vi "Add Pattern Script Header.vi"(8 "error in (no error)":errorcluster, 9 "Pattern Script Frame in":string, 10 "Pattern Name":string, 11 "SPI 4W Pattern Creator in":refnum<class "SPI 4W Pattern Creator.lvclass">) -> (0 "error out":errorcluster, 2 "Pattern Script All out":string, 3 "SPI 4W Pattern Creator out":refnum<class "SPI 4W Pattern Creator.lvclass">)   [LabVIEW 2018, in "SPI 4W Pattern Creator.lvlib" / "SPI 4W Pattern Creator.lvclass"]
uses:
  SPI 4W Pattern Creator.lvclass
  Interfaces/Protocol Interface.lvlibp/Interfaces/Protocol Interface/Pin State.ctl
  Interfaces/Protocol Interface.lvlibp/Interfaces/Protocol Interface/Protocol Interface.lvclass
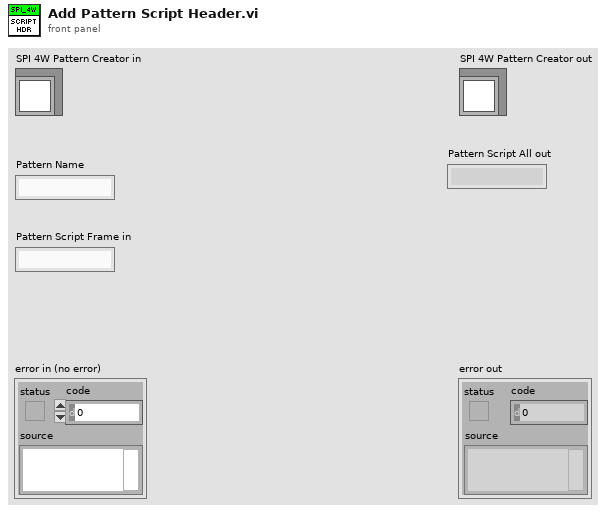
[diagram p1: front panel]
types:
  T1 = typedef "Protocol Interface.lvlibp/Protocol Interface.lvclass/Pin State.ctl" = enum16{"0", "1", "L", "H", "X", "V", "D", "M"}
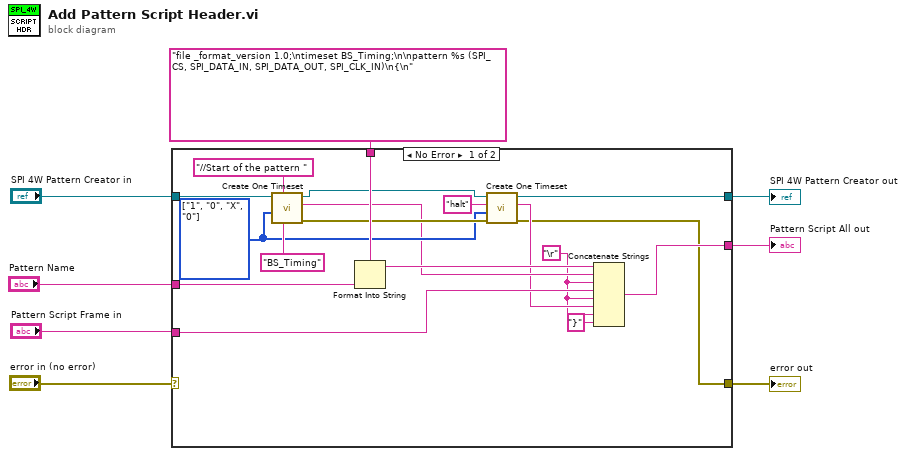
[diagram p0: block diagram]
diagram:
  n1 = case shown="No Error" "error in (no error)" {
    selector: "error in (no error)" -> [_ w28]
    tunnel: "Pattern Name" -> [w26 _]
    tunnel: "file _format_version 1.0;\ntimeset BS_Timing;\n\npattern %s (SPI_CS, SPI_DATA_IN, SPI_DATA_OUT, SPI_CLK_IN)\n{\n" -> [w25 _]
    tunnel: "Pattern Script Frame in" -> [w17 _]
    tunnel: [w13 _] -> w2
    tunnel: [w12 w28] -> w1
    tunnel: "SPI 4W Pattern Creator in" -> [w11 w27]
    tunnel: [w9 w27] -> w3
    frame No Error {
      w15 = "\r"
      w20 = T1[] [enum."1", enum."0", enum."X", enum."0"] items=["0", "1", "L", "H", "X", "V", "D", "M"] ("PinStates")
      n2 = call-dynamic "Create One Timeset.vi"("Timeset Name"="BS_Timing", "Notes"="//Start of the pattern ", "PinStates"=w20, "SPI 4W Pattern Creator in"=w11) -> ("error out"=w22:errorcluster, "String  out"=w18:string, "SPI 4W Pattern Creator out"=w10:refnum<class "SPI 4W Pattern Creator.lvclass">)  [unwired: 5 in]
      n3 = Format Into String(format string=w25, w26) -> (resulting string=w19:string)  [unwired: 2 in, 1 out]
      n4 = call-dynamic "Create One Timeset.vi"("error in (no error)"=w22, "PinStates"=w20, "OpCode"="halt", "SPI 4W Pattern Creator in"=w10) -> ("error out"=w12:errorcluster, "String  out"=w16:string, "SPI 4W Pattern Creator out"=w9:refnum<class "SPI 4W Pattern Creator.lvclass">)  [unwired: 5 in]
      n5 = Concatenate Strings(w19, w18, w15, w17, w15, w16, w15, "}" ("string")) -> (w13:string)
    }
    frame Error {
    }
  }
  "error out" <- w1
  "SPI 4W Pattern Creator out" <- w3
  "Pattern Script All out" <- w2
